vi "n get encoder.vi"(8 "error in (no error)":errorcluster, 9 "zy":i16, 10 "zx":i16, 11 "n":u16) -> (0 "error out":errorcluster, 1 "zy out":i16, 2 "zx out":i16)   [LabVIEW 2015, in "SCANalone4x64.lvlib"]
doc: "__declspec(dllimport) void __stdcall n_get_encoder(unsigned short n, short *zx, short *zy);"
uses:
  <userlib>/SCANalone4x64/SCANalone4x64.lvlib
  <userlib>/SCANalone4x64/SCANalone4x64.dll
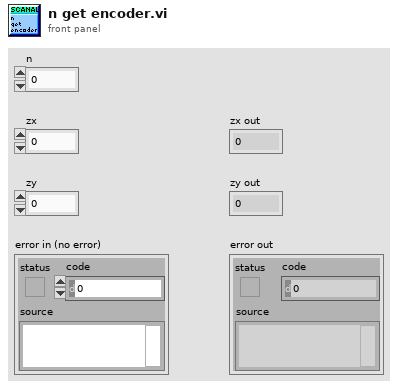
[diagram p1: front panel]
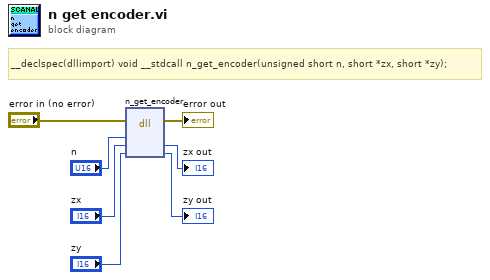
[diagram p0: block diagram]
diagram:
  # "__declspec(dllimport) void __stdcall n_get_encoder(unsigned short n, short *zx, short *zy);"
  n1 = dll-call lib="C:/Program Files/National Instruments/LabVIEW 2015/user.lib/SCANalone4x64/SCANalone4x64.*" fn="n_get_encoder"(error in="error in (no error)", "n"="n", "zx"="zx", "zy"="zy") -> (error out=→"error out":errorcluster, "zx"=→"zx out":i16, "zy"=→"zy out":i16)  [unwired: 4 in, 1 out]
